vi "Get_data.vi"() -> (0 "EOF? and Error status":bool, 1 "Voltage output":dbl[][](graph), 2 "Analogue Binary":i16[][](array[numeric]), 3 "LDA Binary output":u16[][](array[numeric]), 4 "Block Timings":T1={"Started"=0.0, "Ended"=0.0, "Analogue Frequency Hz"=1000.0} {"Analogue Frequency Hz" format="%.2f"}, 5 "PWA Binary":i16[][](array[numeric]), 6 "Block Header":string)   [LabVIEW 2010]
uses:
  Controls/Block_start_and_end.ctl
  Controls/Board_Types.ctl
  Globals/Meas_global.vi
  Globals/LDA_meas_global_1.vi
  Globals/Dynamic_call_global.ph.vi
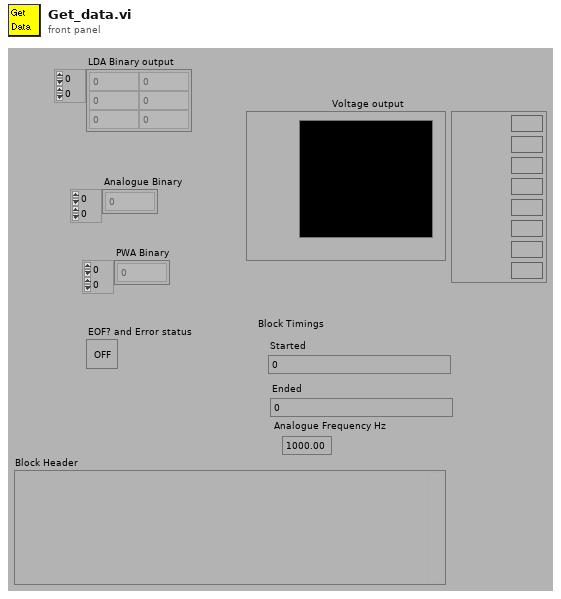
[diagram p1: front panel]
types:
  T1 = typedef "Block_start_and_end.ctl" = cluster{"Started":dbl, "Ended":dbl, "Analogue Frequency Hz":dbl}
  T2 = typedef "Board_Types.ctl" = enum16{"Simulate", "Local ADAM", "Server ADAM", "NI-DAQmx", "NI-DAQmxBase", "ADC488", "DT LV-link"}
  T3 = typedef "Post_Process.ctl" = enum16{"Take New Data", "Post Process Raw Data File"}
  T4 = typedef "PWA_Data.ctl" = enum16{"No PWA Data", "One Ch PWA"}
  T5 = typedef "BSA_Type.ctl" = enum16{"57N11", "BSA F60"}
  T6 = typedef "Ch_and_Spans.ctl" = cluster{"high limit (10V)":sgl, "low limit (-10V)":sgl, "Ch No":i16, "Var name":string, "Use Latest Calib":bool}
  T7 = cluster{"channel":string, "upper input limits":sgl, "lower input limits":sgl, "range":sgl, "polarity":u16, "gain":sgl, "coupling":u16, "input mode":u16, "scale multiplier":dbl, "scale offset":dbl}[]
  T8 = typedef "BSA_info_Cluster.ctl" = cluster{"GPIB Address":string, "No of Check Bytes":i32, "Extra Info":string, "COLOUR":u32, "Wavelength (nm)":dbl}
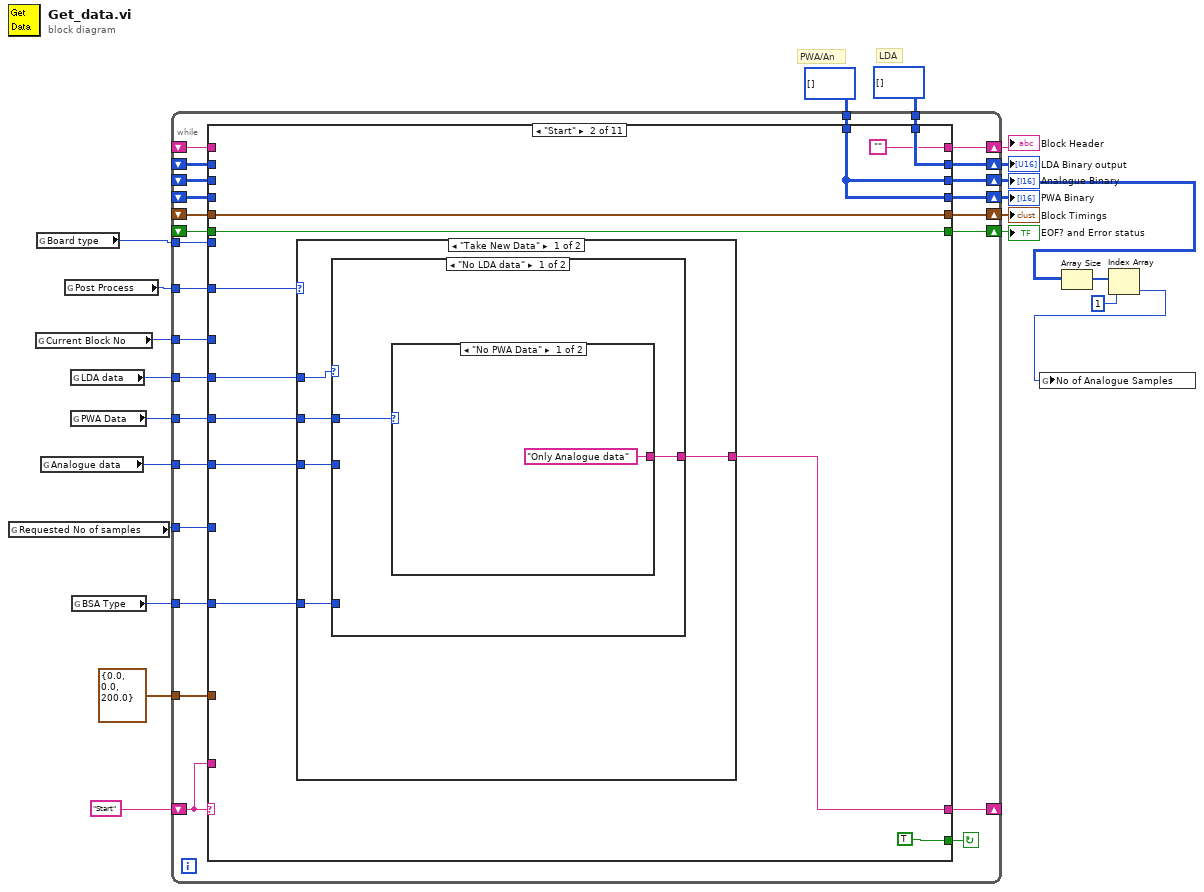
[diagram p0: block diagram]
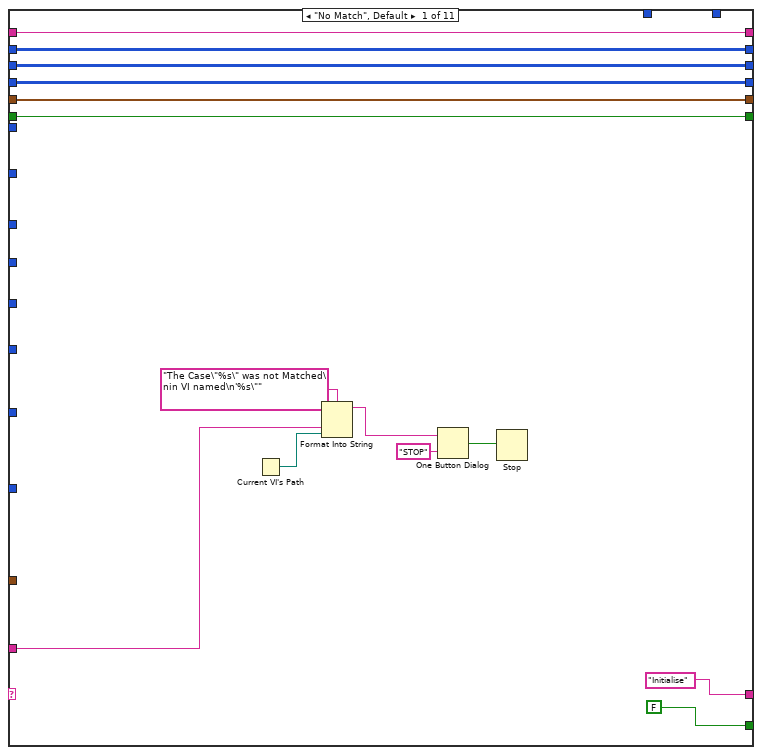
[diagram p2: hidden frame]
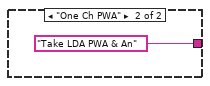
[diagram p3: hidden frame]
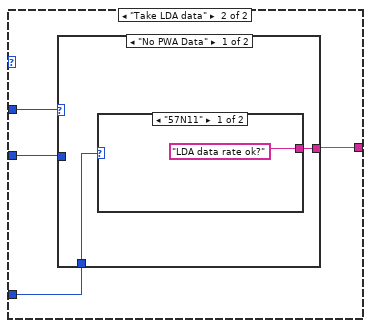
[diagram p4: hidden frame]
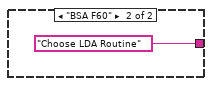
[diagram p5: hidden frame]
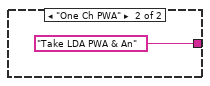
[diagram p6: hidden frame]
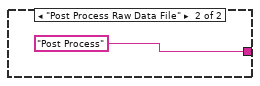
[diagram p7: hidden frame]
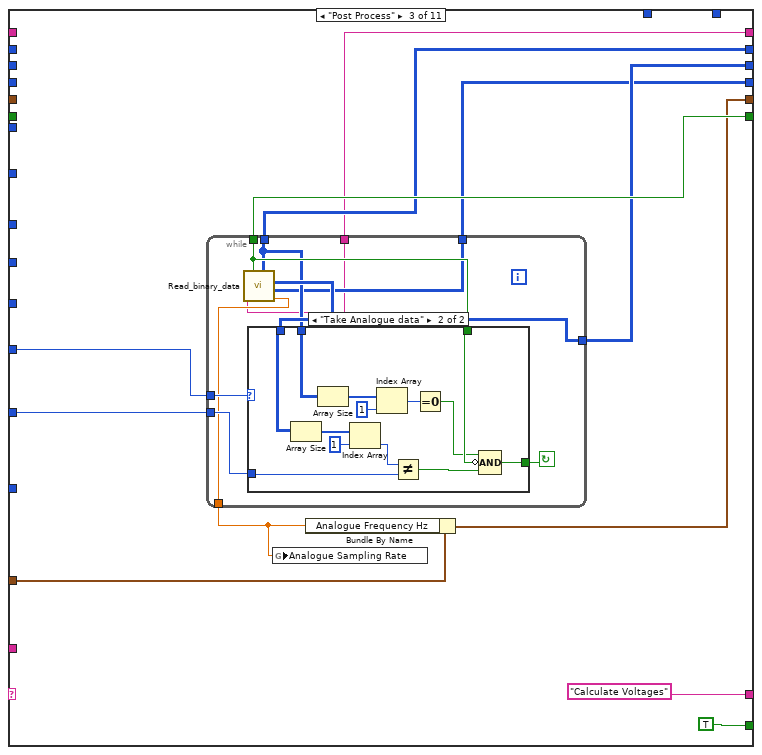
[diagram p8: hidden frame]
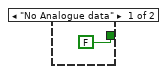
[diagram p9: hidden frame]
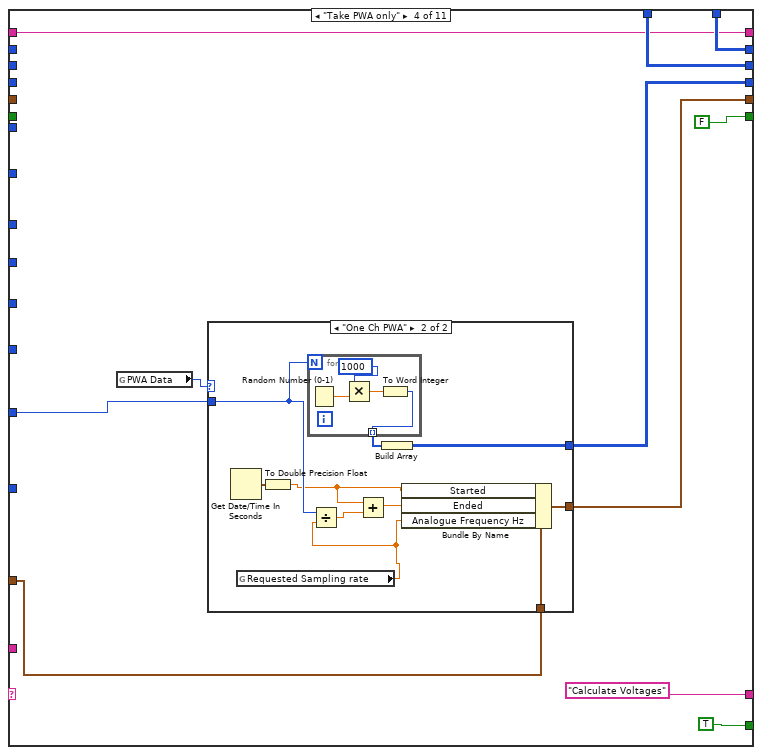
[diagram p10: hidden frame]
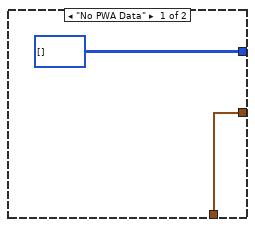
[diagram p11: hidden frame]
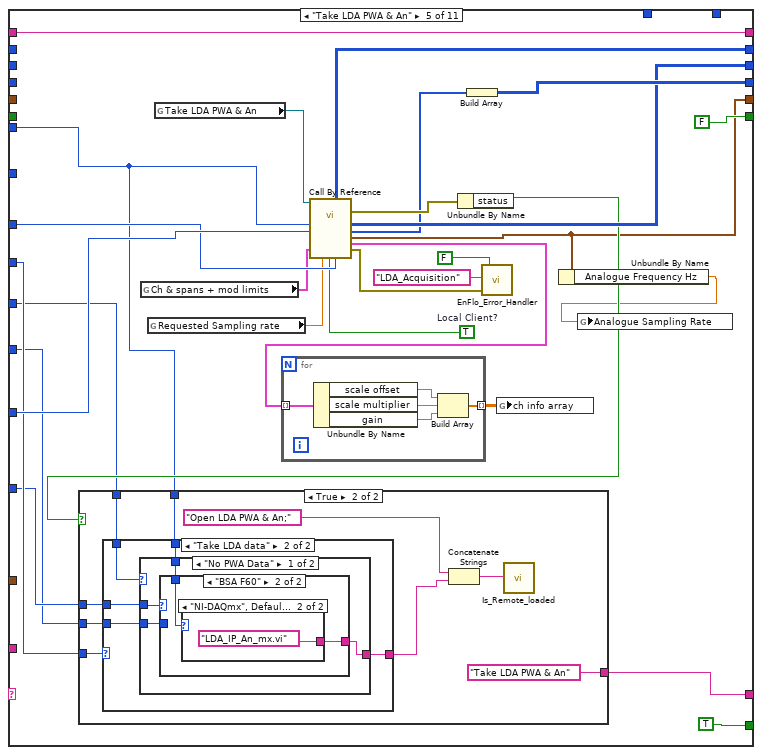
[diagram p12: hidden frame]
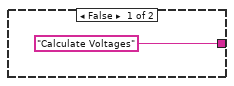
[diagram p13: hidden frame]
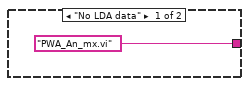
[diagram p14: hidden frame]
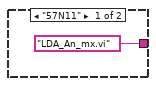
[diagram p15: hidden frame]
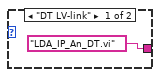
[diagram p16: hidden frame]
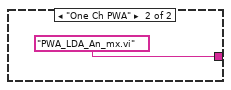
[diagram p17: hidden frame]
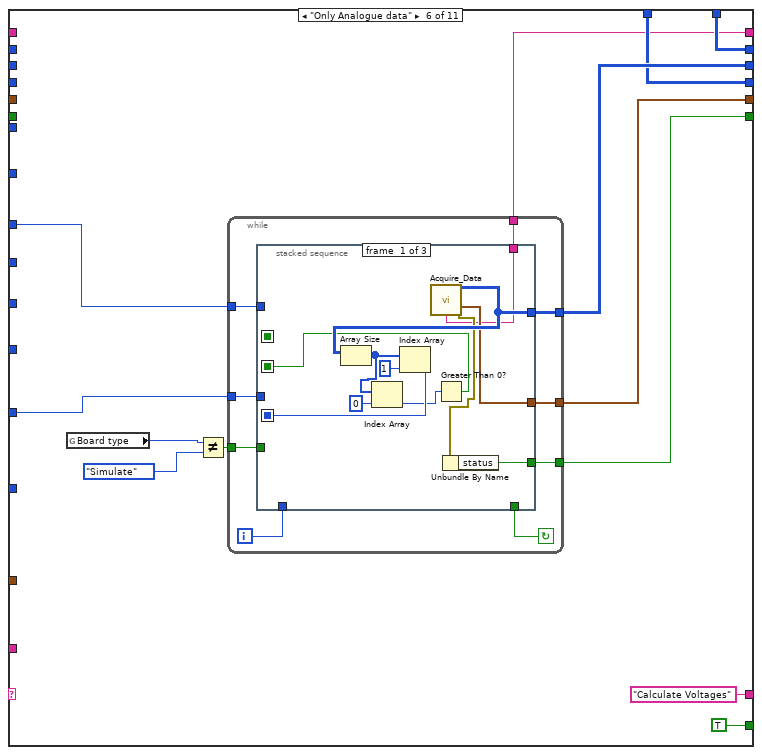
[diagram p18: hidden frame]
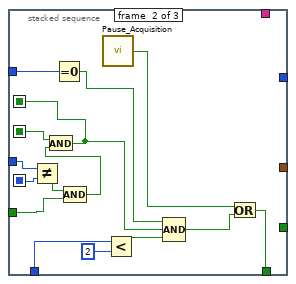
[diagram p19: hidden frame]
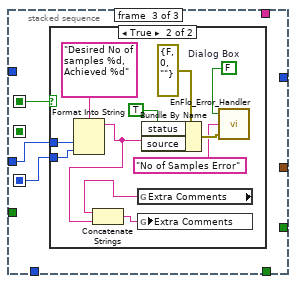
[diagram p20: hidden frame]
diagram:
  # "LDA"
  # "PWA/An"
  n1 = global read "Meas_global.vi" "Requested No of samples"() -> (w14:i32)
  n2 = global read "Meas_global.vi" "Current Block No"() -> (w13:i32)
  n3 = global read "Meas_global.vi" "Board type"() -> (w3:T2)
  n4 = global read "Meas_global.vi" "Analogue data"() -> (w12:enum16{"No Analogue data", "Take Analogue data"})
  n5 = global read "Meas_global.vi" "Post Process"() -> (w15:T3)
  n6 = global read "Meas_global.vi" "LDA data"() -> (w11:enum16{"No LDA data", "Take LDA data"})
  n7 = global read "Meas_global.vi" "PWA Data"() -> (w10:T4)
  n8 = global read "LDA_meas_global_1.vi" "BSA Type"() -> (w1:T5)
  n9 = while {
    shift-left: "Start" -> [w45]
    shift-right: [w46] -> _
    shift-right: [w44] -> w20
    shift-left: _ -> [w43]
    shift-right: [w42] -> w7
    shift-left: _ -> [w41]
    shift-right: [w40] -> w19
    shift-left: _ -> [w39]
    shift-right: [w38] -> w18
    shift-left: _ -> [w37]
    shift-right: [w36] -> w17
    shift-left: _ -> [w35]
    tunnel: T1 {"Started"=0.0, "Ended"=0.0, "Analogue Frequency Hz"=200.0} ("Block Timings") -> [w34]
    tunnel: w15 -> [w33]
    tunnel: w14 -> [w32]
    tunnel: w13 -> [w31]
    tunnel: w12 -> [w30]
    tunnel: w11 -> [w29]
    tunnel: w10 -> [w28]
    tunnel: u16[][] [] ("LDA Binary output") -> [w27]
    tunnel: i16[][] [] ("Analogue Binary output") -> [w26]
    tunnel: w3 -> [w25]
    tunnel: w1 -> [w24]
    shift-right: [w22] -> w2
    shift-left: _ -> [w23]
    stop <- w47 continue-if-true
    n10 = case shown="\"Start\"" w45 {
      tunnel: [FALSE TRUE TRUE TRUE TRUE TRUE TRUE TRUE TRUE w366 FALSE] -> w47
      tunnel: ["Initialise" w69 "Calculate Voltages" "Calculate Voltages" w166 "Calculate Voltages" w279 w329 "Calculate Voltages" "Save Raw Data" "End"] -> w46
      tunnel: w45 -> [w56 _ _ _ _ _ _ _ _ _ _]
      tunnel: [w53 w64 w99 w130 w176 w217 w291 w337 w353 w373 w395] -> w44
      tunnel: w43 -> [w53 _ _ _ _ _ w290 w337 _ w373 w395]
      tunnel: [w52 w65 w98 w129 w178 w222 w288 w336 w352 w372 w394] -> w42
      tunnel: w41 -> [w52 _ _ _ _ _ w289 w336 _ w372 w394]
      tunnel: [w51 w65 w95 w134 w179 w216 w287 w335 w347 w370 w388] -> w40
      tunnel: w39 -> [w51 _ _ _ _ _ w286 w335 _ w370 w388]
      tunnel: [w50 w72 w100 w133 w163 w220 w285 w334 w351 w371 w391] -> w38
      tunnel: w37 -> [w50 w72 _ _ _ _ w284 w334 _ w371 w391]
      tunnel: [w49 w71 w101 FALSE FALSE w221 w283 w333 w350 w369 w396] -> w36
      tunnel: w35 -> [w49 w71 _ _ _ _ w282 w333 _ w369 w396]
      tunnel: w34 -> [_ _ w102 w132 _ _ _ _ _ _ _]
      tunnel: w33 -> [_ w70 _ _ _ _ _ _ _ _ _]
      tunnel: w32 -> [_ _ w97 w135 w181 w224 _ _ _ _ _]
      tunnel: w31 -> [_ _ _ _ w177 w215 w294 _ _ _ w393]
      tunnel: w30 -> [_ w68 w96 _ w159 _ _ w331 _ _ _]
      tunnel: w29 -> [_ w67 _ _ w165 _ _ _ _ _ _]
      tunnel: w28 -> [_ w66 _ _ w164 _ _ _ _ _ _]
      tunnel: w27 -> [_ w64 _ w130 _ w217 _ _ _ _ _]
      tunnel: w26 -> [_ w65 _ w129 _ w216 _ _ w347 _ _]
      tunnel: w25 -> [_ _ _ _ w155 _ _ w332 _ _ _]
      tunnel: w24 -> [_ w63 _ _ w161 _ _ w327 _ _ _]
      tunnel: [w48 "" w93 w128 w160 w214 w276 w328 w346 w364 w387] -> w22
      tunnel: w23 -> [w48 _ _ w128 w160 _ w276 w328 w346 w364 w386]
      frame "No Match", Default {
        n11 = Current VI's Path() -> (path=w55:path)
        n12 = Format Into String(format string="The Case\"%s\" was not Matched\nin VI named\n'%s\"" ("Format String"), w56, w55) -> (resulting string=w59:string)  [unwired: 2 in, 1 out]
        n13 = One Button Dialog(message=w59, button name ("OK")="STOP") -> (true=w57:bool)
        n14 = Stop(stop? (T)=w57) -> ()
      }
      frame "Start" {
        n15 = case shown="\"Take New Data\"" w70 {
          tunnel: [w76 "Post Process"] -> w69
          tunnel: w68 -> [w78 _]
          tunnel: w67 -> [w77 _]
          tunnel: w66 -> [w75 _]
          tunnel: w63 -> [w74 _]
          frame "Take New Data" {
            n16 = case shown="\"No LDA data\"" w77 {
              tunnel: w78 -> [_ w84]
              tunnel: [w79 w86] -> w76
              tunnel: w75 -> [w80 w85]
              tunnel: w74 -> [_ w83]
              frame "No LDA data" {
                n17 = case shown="\"No PWA Data\"" w80 {
                  tunnel: ["Only Analogue data" "Take LDA PWA & An"] -> w79
                  frame "No PWA Data" {
                  }
                  frame "One Ch PWA" {
                  }
                }
              }
              frame "Take LDA data" {
                n18 = case shown="\"No PWA Data\"" w85 {
                  tunnel: [w87 "Take LDA PWA & An"] -> w86
                  tunnel: w84 -> [_ _]
                  tunnel: w83 -> [w88 _]
                  frame "No PWA Data" {
                    n19 = case shown="\"57N11\"" w88 {
                      tunnel: ["LDA data rate ok?" "Choose LDA Routine"] -> w87
                      frame "57N11" {
                      }
                      frame "BSA F60" {
                      }
                    }
                  }
                  frame "One Ch PWA" {
                  }
                }
              }
            }
          }
          frame "Post Process Raw Data File" {
          }
        }
      }
      frame "Post Process" {
        n20 = while {
          tunnel: [w107] -> w94
          tunnel: w96 -> [w109]
          tunnel: w97 -> [w110]
          tunnel: [w112] -> w101
          tunnel: [w108] -> w99
          tunnel: [w113] -> w98
          tunnel: [w106] -> w95
          tunnel: [w105] -> w93
          stop <- w111 continue-if-true
          n21 = call "Read_binary_data.vi"() -> ("Analogue Frequency Hz"=w107:dbl, "PWA Binary"=w106:i16[][], "Analogue Binary"=w113:i16[][], "LDA Binary output"=w108:u16[][], "EOF?"=w112:bool, "Block Header"=w105:string)  [unwired: 4 out]
          n22 = case shown="\"Take Analogue data\"" w109 {
            tunnel: w113 -> [_ w124]
            tunnel: w112 -> [_ w122]
            tunnel: [FALSE w121] -> w111
            tunnel: w110 -> [_ w120]
            tunnel: w108 -> [_ w117]
            frame "No Analogue data" {
            }
            frame "Take Analogue data" {
              n23 = Array Size(array=w124) -> (size(s)=w126:i32[])
              n24 = Array Size(array=w117) -> (size(s)=w119:i32[])
              n25 = Index Array(array=w126, index=1 ("Index")) -> (element=w125:i32)
              n26 = Index Array(array=w119, index=1 ("Index")) -> (element=w116:i32)
              n27 = Not Equal?(x=w125, y=w120) -> (x != y?=w123:bool)
              n28 = Equal To 0?(x=w116) -> (x = 0?=w115:bool)
              n29 = Compound Arithmetic op=AND(w115, invert w122, w123) -> (w121:bool)
            }
          }
        }
        n30 = global write "Meas_global.vi" "Analogue Sampling Rate"(w94) -> ()
        n31 = Bundle By Name(cluster=w102, "Analogue Frequency Hz"=w94) -> (w100:T1)
      }
      frame "Take PWA only" {
        n32 = global read "Meas_global.vi" "PWA Data"() -> (w136:T4)
        n33 = case shown="\"One Ch PWA\"" w136 {
          tunnel: w135 -> [_ w147]
          tunnel: [i16[][] [] w149] -> w134
          tunnel: [w139 w143] -> w133
          tunnel: w132 -> [w139 w142]
          frame "No PWA Data" {
          }
          frame "One Ch PWA" {
            n34 = Get Date/Time In Seconds() -> (seconds since 1Jan1904=w148:timestamp)
            n35 = global read "Meas_global.vi" "Requested Sampling rate"() -> (w146:dbl)
            n36 = To Double Precision Float(number=w148) -> (double precision float=w144:dbl)
            n37 = for {
              N: w147 -> [_]
              tunnel: [w151] -> w150 mode=indexing
              n38 = Random Number (0-1)() -> (number: 0 to 1=w154:dbl)
              n39 = Multiply(x=1000, y=w154) -> (x*y=w152:dbl)
              n40 = To Word Integer(number=w152) -> (16bit integer=w151:i16)
            }
            n41 = Divide(x=w147, y=w146) -> (x/y=w145:dbl)
            n42 = Add(x=w144, y=w145) -> (x+y=w141:dbl)
            n43 = Build Array(w150) -> (w149:i16[][])
            n44 = Bundle By Name(cluster=w142, "Started"=w144, "Ended"=w141, "Analogue Frequency Hz"=w146) -> (w143:T1)
          }
        }
      }
      frame "Take LDA PWA & An" {
        w172 = TRUE  # Local Client?
        n45 = global read "Meas_global.vi" "Ch & spans + mod limits"() -> (w175:T6[])
        n46 = global read "Meas_global.vi" "Requested Sampling rate"() -> (w171:dbl)
        n47 = global read "Dynamic_call_global.ph.vi" "Take LDA PWA & An"() -> (w170:refnum<vi>)
        n48 = call-by-ref "?"(reference=w170, "Board type"=w155, "No of LDA samples"=w181, "Ch & spans"=w175, "LDA Sampling rate (Hz)"=w171, "Local Client?"=w172, "Current Block No"=w177) -> (error out=w169:errorcluster, "LDA Binary output"=w176:u16[][], "I16 Analogue data block"=w178:i16[][], "I16 TOF block (mu.s)"=w168:i16[], "Block Timings"=w163:T1, "group channel settings"=w174:T7, 15:"error out"=w157:errorcluster)  [unwired: 5 in, 1 out]
        n49 = for {
          tunnel: w174 -> [w213] mode=indexing
          tunnel: [w209] -> w173 mode=indexing
          n50 = Unbundle By Name(w213) -> ("scale offset"=w212:dbl, "scale multiplier"=w211:dbl, "gain"=w210:sgl)
          n51 = Build Array(w212, w211, w210) -> (w209:dbl[])
        }
        n52 = Unbundle By Name(w169) -> ("status"=w167:bool)
        n53 = case shown="True" w167 {
          tunnel: ["Calculate Voltages" "Take LDA PWA & An"] -> w166
          tunnel: w165 -> [_ w188]
          tunnel: w164 -> [_ w187]
          tunnel: w161 -> [_ w186]
          tunnel: w159 -> [_ w185]
          tunnel: w155 -> [_ w184]
          frame False {
          }
          frame True {
            n54 = case shown="\"Take LDA data\"" w188 {
              tunnel: ["PWA_An_mx.vi" ("name or relative path") w198] -> w189
              tunnel: w187 -> [_ w197]
              tunnel: w186 -> [_ w196]
              tunnel: w185 -> [_ w195]
              tunnel: w184 -> [_ w194]
              frame "No LDA data" {
              }
              frame "Take LDA data" {
                n55 = case shown="\"No PWA Data\"" w197 {
                  tunnel: [w201 "PWA_LDA_An_mx.vi" ("name or relative path")] -> w198
                  tunnel: w196 -> [w202 _]
                  tunnel: w195 -> [w200 _]
                  tunnel: w194 -> [w199 _]
                  frame "No PWA Data" {
                    n56 = case shown="\"BSA F60\"" w202 {
                      tunnel: ["LDA_An_mx.vi" ("name or relative path") w205] -> w201
                      tunnel: w200 -> [_ _]
                      tunnel: w199 -> [_ w204]
                      frame "57N11" {
                      }
                      frame "BSA F60" {
                        n57 = case shown="\"NI-DAQmx\", Default" w204 {
                          tunnel: ["LDA_IP_An_DT.vi" ("name or relative path") "LDA_IP_An_mx.vi" ("name or relative path")] -> w205
                          frame "DT LV-link" {
                          }
                          frame "NI-DAQmx", Default {
                          }
                        }
                      }
                    }
                  }
                  frame "One Ch PWA" {
                  }
                }
              }
            }
            n58 = Concatenate Strings("Open LDA PWA & An;", w189) -> (w190:string)
            n59 = call "Is_Remote_loaded.vi"("Sub VI to call"=w190) -> ()
          }
        }
        n60 = Build Array(w168) -> (w179:i16[][])
        n61 = call "EnFlo_Error_Handler.vi"("error in (no error)"=w157, "Error Type"="LDA_Acquisition", "Dialog Box (T)"=FALSE) -> ()  [unwired: 3 out]
        n62 = global write "Meas_global.vi" "ch info array"(w173) -> ()
        n63 = Unbundle By Name(w163) -> ("Analogue Frequency Hz"=w162:dbl)
        n64 = global write "Meas_global.vi" "Analogue Sampling Rate"(w162) -> ()
      }
      frame "Only Analogue data" {
        n65 = global read "Meas_global.vi" "Board type"() -> (w226:T2)
        n66 = Not Equal?(x=w226, y=Board_Types."Simulate" ("Board type")) -> (x != y?=w223:bool)
        n67 = while {
          tunnel: w224 -> [w235]
          tunnel: w223 -> [w234]
          tunnel: [w233] -> w222
          tunnel: [w231] -> w221
          tunnel: [w230] -> w220
          tunnel: w215 -> [w228]
          tunnel: [w227] -> w214
          i -> [w229]
          stop <- w232 continue-if-true
          n68 = stacked-sequence {
            seq-local: [w244 _ _] -> [_ w261 w262]
            seq-local: [_ w252 _] -> [_ _ w264]
            seq-local: [w239 _ _] -> [_ w259 _]
            tunnel: [_ w249 _] -> w232
            tunnel: [w245 _ _] -> w233
            tunnel: w235 -> [_ w260 w263]
            tunnel: [w243 _ _] -> w230
            tunnel: [w237 _ _] -> w231
            tunnel: w234 -> [_ w256 _]
            tunnel: w229 -> [_ w255 _]
            tunnel: w228 -> [_ w248 _]
            tunnel: [w236 _ _] -> w227
            frame #0 {
              n69 = call "Acquire_Data.vi"() -> ("Binary output"=w245:i16[][], "Block Timings"=w243:T1, "Add to Block Header"=w236:string, "error out"=w238:errorcluster)  [unwired: 12 out]
              n70 = Array Size(array=w245) -> (size(s)=w242:i32[])
              n71 = Index Array(array=w242, index=0) -> (element=w240:i32)
              n72 = Index Array(array=w242, index=1 ("Index")) -> (element=w244:i32)
              n73 = Greater Than 0?(x=w240) -> (x > 0?=w239:bool)
              n74 = Unbundle By Name(w238) -> ("status"=w237:bool)
            }
            frame #1 {
              n75 = Not Equal?(x=w260, y=w261) -> (x != y?=w258:bool)
              n76 = Equal To 0?(x=w248) -> (x = 0?=w247:bool)
              n77 = Compound Arithmetic op=AND(w258, w256) -> (w257:bool)
              n78 = And(x=w259, y=w257) -> (x .and. y?=w252:bool)
              n79 = call "Pause_Acquisition.vi"() -> ("Paused"=w251:bool)
              n80 = Less?(x=w255, y=2) -> (x < y?=w253:bool)
              n81 = Compound Arithmetic op=AND(w247, w252, w253) -> (w250:bool)
              n82 = Or(x=w251, y=w250) -> (x .or. y?=w249:bool)
            }
            frame #2 {
              n83 = case shown="True" w264 {
                tunnel: w263 -> [_ w272]
                tunnel: w262 -> [_ w271]
                frame False {
                }
                frame True {
                  w273 = FALSE  # Dialog Box
                  n84 = Format Into String(format string="Desired No of samples %d, Achieved %d" ("Format String"), w272, w271) -> (resulting string=w266:string)  [unwired: 2 in, 1 out]
                  n85 = global read "Meas_global.vi" "Extra Comments"() -> (w267:string)
                  n86 = Concatenate Strings(w267, w266) -> (w265:string)
                  n87 = global write "Meas_global.vi" "Extra Comments"(w265) -> ()
                  n88 = Bundle By Name(cluster=errorcluster {"status"=FALSE, "code"=0, "source"=""} ("error in (no error)"), "status"=TRUE ("Bundle Element"), "source"=w266) -> (w274:errorcluster)
                  n89 = call "EnFlo_Error_Handler.vi"("error in (no error)"=w274, "Error Type"="No of Samples Error", "Dialog Box (T)"=w273) -> ()  [unwired: 3 out]
                }
              }
            }
          }
        }
      }
      frame "LDA data rate ok?" {
        n90 = while {
          tunnel: [w317] -> w293 mode=indexing
          tunnel: [w319] -> w280
          i -> [w322]
          stop <- w318 continue-if-true
          n91 = global read "LDA_meas_global_1.vi" "BSA1 info"() -> (w325:T8)
          n92 = Unbundle By Name(w325) -> ("GPIB Address"=w324:string)
          n93 = Less?(x=w322, y=8) -> (x < y?=w320:bool)
          n94 = call "data_rate.vi"("GPIB address"=w324) -> ("Data rate (Hz)"=w317:dbl)
          n95 = Greater?(x=w317, y=5.0) -> (0:w319:bool)
          n96 = Compound Arithmetic op=AND(invert w319, w320) -> (w318:bool)
          n97 = case shown="True" w318 {
            frame False {
            }
            frame True {
              n98 = Wait Until Next ms Multiple(millisecond multiple=u32 1000) -> ()  [unwired: 1 out]
            }
          }
        }
        n99 = Array Max & Min(array=w293) -> (max value=w292:dbl)  [unwired: 3 out]
        n100 = case shown="True" w280 {
          tunnel: w294 -> [_ w312]
          tunnel: w292 -> [w296 w311]
          tunnel: [u16[][] [] ("LDA Binary output") w310] -> w291
          tunnel: w290 -> [_ w310]
          tunnel: w289 -> [_ w309]
          tunnel: [i16[][] [] ("Binary output") w309] -> w288
          tunnel: [w303 w308] -> w287
          tunnel: w286 -> [w303 w308]
          tunnel: [T1 {"Started"=0.0, "Ended"=0.0, "Analogue Frequency Hz"=200.0} ("Block Timings") w307] -> w285
          tunnel: w284 -> [_ w307]
          tunnel: [TRUE w306] -> w283
          tunnel: w282 -> [_ w306]
          frame False {
            n101 = Number To Fractional String(number=w296, precision (6)=1) -> (F-format string=w298:string)  [unwired: 2 out]
            n102 = Concatenate Strings("BSA data rate is ", w298, " Hz.") -> (w301:string)
            n103 = global write "Meas_global.vi" "BSA data rate string"(w301) -> ()
          }
          frame True {
            n104 = Greater?(x=w312, y=1) -> (0:w314:bool)
            n105 = global read "Meas_global.vi" "LDA frequency"() -> (w316:dbl)
            n106 = Select(t=w316, s=w314, f=w311) -> (s? t:f=w313:dbl)
            n107 = global write "Meas_global.vi" "Actual Sampling rate (Hz)"(w313) -> ()
          }
        }
        n108 = Select(t="Choose LDA Routine", s=w280, f="Calculate Voltages") -> (s? t:f=w279:string)
      }
      frame "Choose LDA Routine" {
        n109 = case shown="\"Take Analogue data\"" w331 {
          tunnel: [w339 w343] -> w329
          tunnel: w332 -> [_ w342]
          tunnel: w327 -> [w338 _]
          frame "No Analogue data" {
            n110 = case shown="\"BSA F60\"" w338 {
              tunnel: ["Take LDA+Analogue data" "Take LDA PWA & An"] -> w339
              frame "57N11" {
              }
              frame "BSA F60" {
              }
            }
          }
          frame "Take Analogue data" {
            n111 = case shown="\"NI-DAQmx\", Default" w342 {
              tunnel: ["Take LDA PWA & An" "Take LDA+Analogue data"] -> w343
              frame "NI-DAQmx", Default {
              }
              frame "ADC488" {
              }
            }
          }
        }
      }
      frame "Take LDA+Analogue data" {
        n112 = while {
          tunnel: [w354] -> w350
          tunnel: [w355] -> w351
          tunnel: [w357] -> w353
          tunnel: [w356] -> w352
          i -> [w358]
          stop <- w359 continue-if-true
          n113 = Less?(x=w358, y=1) -> (x < y?=w362:bool)
          n114 = call "Get_LDA_+_An_data.vi"("Try number"=w358) -> ("LDA Binary output"=w357:u16[][], "Analogue Binary output"=w356:i16[][], "Block Timings"=w355:T1, "Repeat Block"=w354:bool)
          n115 = And(x=w354, y=w362) -> (x .and. y?=w361:bool)
          n116 = call "Pause_Acquisition.vi"() -> ("Paused"=w360:bool)
          n117 = Or(x=w360, y=w361) -> (x .or. y?=w359:bool)
        }
      }
      frame "Calculate Voltages" {
        n118 = global read "Meas_global.vi" "ch info array"() -> (w374:dbl[][])
        n119 = global read "Meas_global.vi" "Raw data option"() -> (w368:enum16{"Save raw data", "Raw data not saved"})
        n120 = for {
          tunnel: [w377] -> w365 mode=indexing
          tunnel: w372 -> [w384] mode=indexing
          tunnel: w374 -> [w380] mode=indexing
          n121 = To Double Precision Float(number=w384) -> (double precision float=w383:dbl[])
          n122 = Index Array(array=w380, index=0) -> (element=w379:dbl)
          n123 = Index Array(array=w380, index=1) -> (element=w378:dbl)
          n124 = Multiply(x=w383, y=w378) -> (x*y=w385:dbl[])
          n125 = Add(x=w379, y=w385) -> (x+y=w377:dbl[])
        }
        "Voltage output" <- w365
        n126 = case shown="\"Raw data not saved\"" w368 {
          tunnel: [TRUE FALSE] -> w366
          frame "Save raw data" {
          }
          frame "Raw data not saved" {
          }
        }
      }
      frame "Save Raw Data" {
        n127 = Greater Than 0?(x=w393) -> (x > 0?=w392:bool)
        n128 = call "Save_Raw_data.vi"("Add to Block Header"=w386, "PWA Binary"=w388, "Analogue Binary"=w394, "append to file? (new file:F)"=w392, "Block Timings"=w391, "LDA Binary"=w395) -> ("Block Header"=w387:string)  [unwired: 3 in]
      }
    }
  }
  "EOF? and Error status" <- w17
  "LDA Binary output" <- w20
  "Analogue Binary" <- w7
  "PWA Binary" <- w19
  "Block Timings" <- w18
  "Block Header" <- w2
  n129 = Array Size(array=w7) -> (size(s)=w6:i32[])
  n130 = Index Array(array=w6, index=1) -> (element=w4:i32)
  n131 = global write "Meas_global.vi" "No of Analogue Samples"(w4) -> ()
